vi "Compressor Oper.vi"   [LabVIEW 2016]
uses:
  Robot Global Data.vi
  <vilib>/Rock Robotics/WPI/Utilities/WPI_GetSetVariantRefNum.vi
types:
  T1 = typedef "WPI_DriverStationRobotMode2.ctl" = enum16{"Autonomous Disabled", "Autonomous Enabled", "Teleop Disabled", "Teleop Enabled", "Disconnected", "Finish", "Test Disabled", "Test Enabled", "Emergency Stopped"}
  T2 = typedef "WPI_CompressorDevRef.ctl" = cluster{"DevStatus":errorcluster, "Pneumatics Control Module":u8}
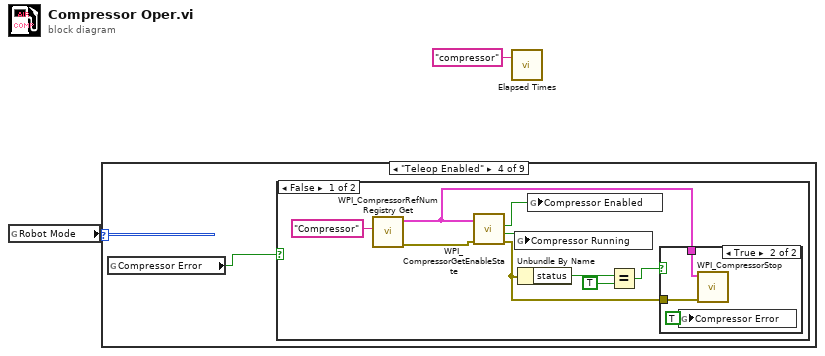
[diagram p0: block diagram]
diagram:
  n1 = global read "Robot Global Data.vi" "Robot Mode"() -> (w2:T1)
  n2 = case shown="\"Teleop Enabled\"" w2 {
    frame "Autonomous Disabled", Default {
    }
    frame "Autonomous Enabled" {
    }
    frame "Teleop Disabled" {
    }
    frame "Teleop Enabled" {
      n3 = global read "Robot Global Data.vi" "Compressor Error"() -> (w3:bool)
      n4 = case shown="False" w3 {
        frame False {
          n5 = call <vilib>:"WPI_CompressorRefNum Registry Get.vi"("refnum name"="Compressor") -> ("error out"=w11:errorcluster, "CompressorDevRef"=w5:T2)  [unwired: 9 in]
          n6 = call <vilib>:"WPI_CompressorGetEnableState.vi"("error in (no error)"=w11, "CompressorDevRef"=w5) -> ("error out"=w4:errorcluster, "Compressor Running"=w10:bool, "Enabled"=w9:bool)  [unwired: 6 in, 1 out]
          n7 = global write "Robot Global Data.vi" "Compressor Running"(w10) -> ()
          n8 = Unbundle By Name(w4) -> ("status"=w8:bool)
          n9 = global write "Robot Global Data.vi" "Compressor Enabled"(w9) -> ()
          n10 = Equal?(x=w8, y=TRUE) -> (x = y?=w6:bool)
          n11 = case shown="True" w6 {
            tunnel: w5 -> [_ w14]
            tunnel: w4 -> [_ w13]
            frame False {
            }
            frame True {
              n12 = global write "Robot Global Data.vi" "Compressor Error"(TRUE ("Compressor Error")) -> ()
              n13 = call <vilib>:"WPI_CompressorStop.vi"("error in (no error)"=w13, "CompressorDevRef"=w14) -> ()  [unwired: 8 in, 2 out]
            }
          }
        }
        frame True {
        }
      }
    }
    frame "Disconnected" {
    }
    frame "Finish" {
    }
    frame "Test Disabled" {
    }
    frame "Test Enabled" {
    }
    frame "Emergency Stopped" {
    }
  }
  n14 = call "Elapsed Times.vi"("Call Name"="compressor") -> ()  [unwired: 2 in, 1 out]
